vi "PolyRoots.vi"(0 "P":cluster{"x":dbl, "y":dbl, "z":dbl}={"x"=-4.0, "y"=0.0, "z"=4.0} {"x" format="%.2f"; "z" format="%.2f"; "y" format="%.2f"}, 11 "phi":dbl format="%.2f", 12 "constant":dbl format="%.2f", 13 "theta lim":dbl format="%.2f") -> (4 "Polynomial Roots":dbl[](array[numeric]) format="%.2f")   [LabVIEW 2022 SP3]
uses:
  <vilib>/Analysis/polynomials.llb/Polynomial Roots (DBL).vi
  <vilib>/Analysis/NI_AALPro.lvlib
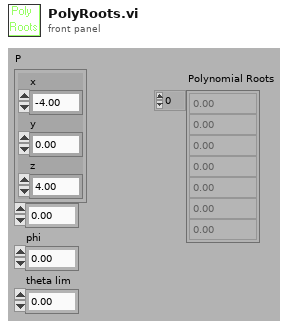
[diagram p1: front panel]
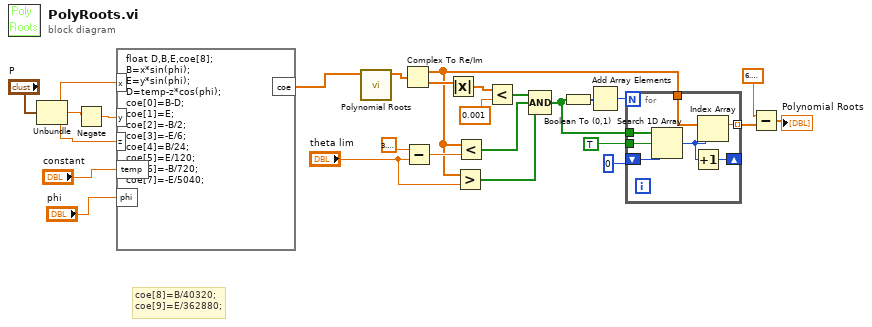
[diagram p0: block diagram]
diagram:
  # "coe[8]=B/40320;\ncoe[9]=E/362880;"
  n1 = Unbundle("P") -> ("x"=w3:dbl, "y"=w2:dbl, "z"=w1:dbl)
  n2 = Negate(x=w2) -> (-x=w20:dbl)
  n3 = formula code="float D,B,E,coe[8];\nB=x*sin(phi);\nE=y*sin(phi);\nD=temp-z*cos(phi);\ncoe[0]=B-D;\ncoe[1]=E;\ncoe[2]=-B/2;\ncoe[3]=-E/6;\ncoe[4]=B/24;\ncoe[5]=E/120;\ncoe[6]=-B/720;\ncoe[7]=-E/5040;"("x"=w3, "y"=w20, "z"=w1, "temp"="constant", "phi"="phi") -> ("coe"=w16:dbl[])
  n4 = call-poly <vilib>:"Polynomial Roots.vi"("P(x)"=w16) -> ("Roots"=w22:cdb[])  [unwired: 1 in, 9 out]
  n5 = Complex To Re/Im(x + iy=w22) -> (x=w7:dbl[], y=w14:dbl[])
  n6 = Subtract(x=3.141592653589793, y="theta lim") -> (x-y=w11:dbl)
  n7 = Absolute Value(x=w14) -> (abs(x)=w12:dbl[])
  n8 = Greater?(x=w7, y="theta lim") -> (0:w8:bool[])
  n9 = Less?(x=w7, y=w11) -> (x < y?=w9:bool[])
  n10 = Less?(x=w12, y=0.001) -> (x < y?=w15:bool[])
  n11 = Compound Arithmetic op=AND(w15, w9, w8) -> (w6:bool[])
  n12 = Boolean To (0,1)(Boolean=w6) -> (0, 1=w25:i16[])
  n13 = Add Array Elements(numeric array=w25) -> (sum=w5:i16)
  n14 = for {
    N: w5 -> [_]
    tunnel: w6 -> [w34]
    tunnel: TRUE -> [w33]
    tunnel: w7 -> [w32]
    tunnel: [w31] -> w19 mode=indexing
    shift-right: [w28] -> _
    shift-left: 0 -> [w29]
    n15 = Search 1D Array(1D array=w34, element=w33, start index (0)=w29) -> (index of element=w30:i32)
    n16 = Increment(x=w30) -> (x+1=w28:i32)
    n17 = Index Array(array=w32, index=w30) -> (element=w31:dbl)
  }
  n18 = Subtract(x=6.283185307179586, y=w19) -> (x-y=→"Polynomial Roots":dbl[])
